vi "Day 10.vi"() -> ()   [LabVIEW 2023]
panel:
  out "Answer 2":bool[][](array[boolean])
  out "Answer 1":i32
  in  "test":bool
  in  "test input":string="addx 15\naddx -11\naddx 6\naddx -3\naddx 5\naddx -1\naddx -8\naddx 13\naddx 4\nnoop\naddx -1\naddx 5\naddx -1\naddx 5\naddx -1\naddx 5\naddx -1\naddx 5\naddx -1\naddx -35\naddx 1\naddx 24\naddx -19\naddx 1\naddx 16\naddx -11\nnoop\nnoop\naddx 21\naddx -15\nnoop\nnoop\naddx -3\naddx 9\naddx 1\naddx -3\naddx 8\naddx 1\naddx 5\nnoop\nnoop\nnoop\nnoop\nnoop\naddx -36\nnoop\naddx 1\naddx 7\nnoop\nnoop\nnoop\naddx 2\naddx 6\nnoop\nnoop\nnoop\nnoop\nnoop\naddx 1\nnoop\nnoop\naddx 7\naddx 1\nnoop\naddx -13\naddx 13\naddx 7\nnoop\naddx 1\naddx -33\nnoop\nnoop\nnoop\naddx 2\nnoop\nnoop\nnoop\naddx 8\nnoop\naddx -1\naddx 2\naddx 1\nnoop\naddx 17\naddx -9\naddx 1\naddx 1\naddx -3\naddx 11\nnoop\nnoop\naddx 1\nnoop\naddx 1\nnoop\nnoop\naddx -13\naddx -19\naddx 1\naddx 3\naddx 26\naddx -30\naddx 12\naddx -1\naddx 3\naddx 1\nnoop\nnoop\nnoop\naddx -9\naddx 18\naddx 1\naddx 2\nnoop\nnoop\naddx 9\nnoop\nnoop\nnoop\naddx -1\naddx 2\naddx -37\naddx 1\naddx 3\nnoop\naddx 15\naddx -21\naddx 22\naddx -6\naddx 1\nnoop\naddx 2\naddx 1\nnoop\naddx -10\nnoop\nnoop\naddx 20\naddx 1\naddx 2\naddx 2\naddx -6\naddx -11\nnoop\nnoop\nnoop"
  in  "input":string="noop\nnoop\nnoop\naddx 3\naddx 20\nnoop\naddx -12\nnoop\naddx 4\nnoop\nnoop\nnoop\naddx 1\naddx 2\naddx 5\naddx 16\naddx -14\naddx -25\naddx 30\naddx 1\nnoop\naddx 5\nnoop\naddx -38\nnoop\nnoop\nnoop\naddx 3\naddx 2\nnoop\nnoop\nnoop\naddx 5\naddx 5\naddx 2\naddx 13\naddx 6\naddx -16\naddx 2\naddx 5\naddx -15\naddx 16\naddx 7\nnoop\naddx -2\naddx 2\naddx 5\naddx -39\naddx 4\naddx -2\naddx 2\naddx 7\nnoop\naddx -2\naddx 17\naddx -10\nnoop\nnoop\naddx 5\naddx -1\naddx 6\nnoop\naddx -2\naddx 5\naddx -8\naddx 12\naddx 3\naddx -2\naddx -19\naddx -16\naddx 2\naddx 5\nnoop\naddx 25\naddx 7\naddx -29\naddx 3\naddx 4\naddx -4\naddx 9\nnoop\naddx 2\naddx -20\naddx 23\naddx 1\nnoop\naddx 5\naddx -10\naddx 14\naddx 2\naddx -1\naddx -38\nnoop\naddx 20\naddx -15\nnoop\naddx 7\nnoop\naddx 26\naddx -25\naddx 2\naddx 7\nnoop\nnoop\naddx 2\naddx -5\naddx 6\naddx 5\naddx 2\naddx 8\naddx -3\nnoop\naddx 3\naddx -2\naddx -38\naddx 13\naddx -6\nnoop\naddx 1\naddx 5\nnoop\nnoop\nnoop\nnoop\naddx 2\nnoop\nnoop\naddx 7\naddx 3\naddx -2\naddx 2\naddx 5\naddx 2\nnoop\naddx 1\naddx 5\nnoop\nnoop\nnoop\nnoop\nnoop\nnoop\n"
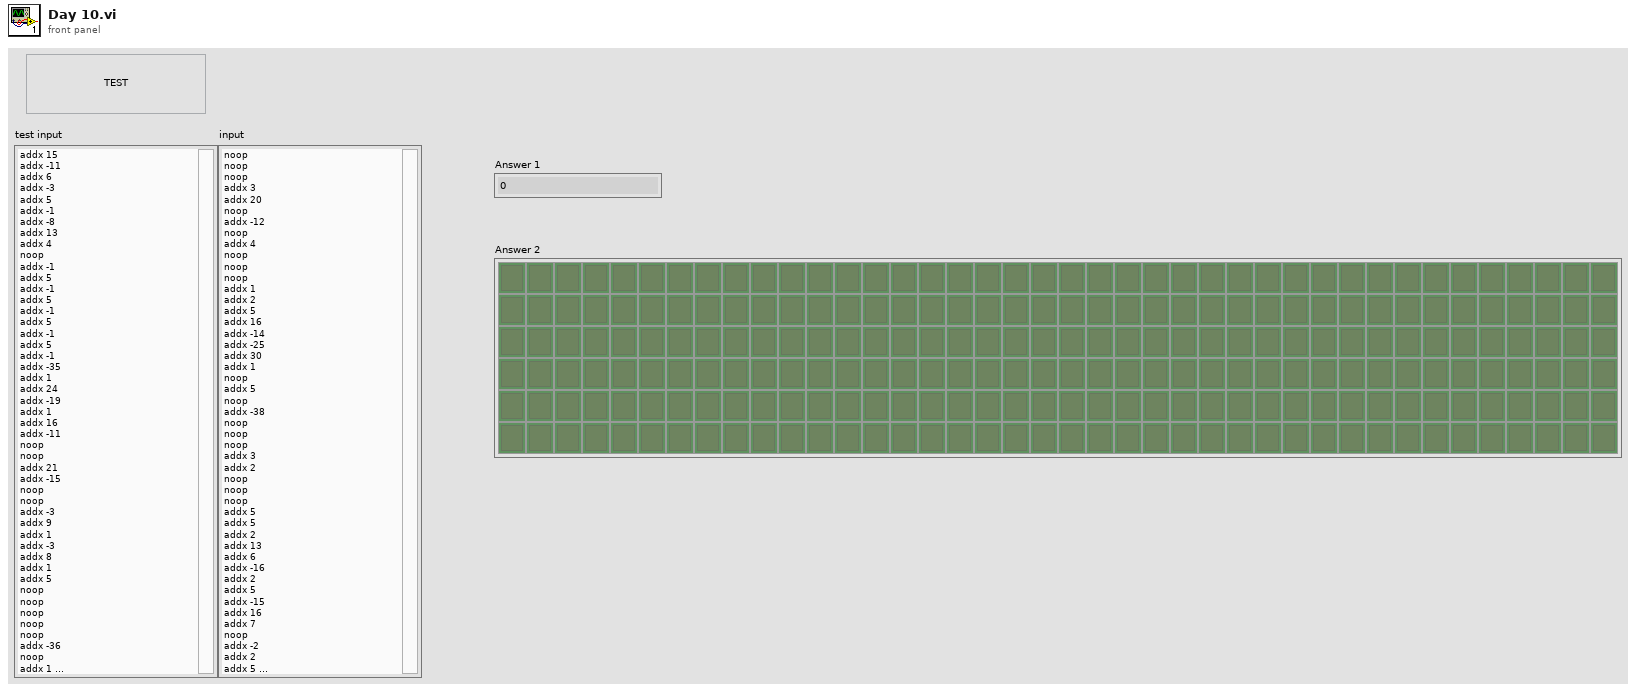
[diagram p1: front panel]
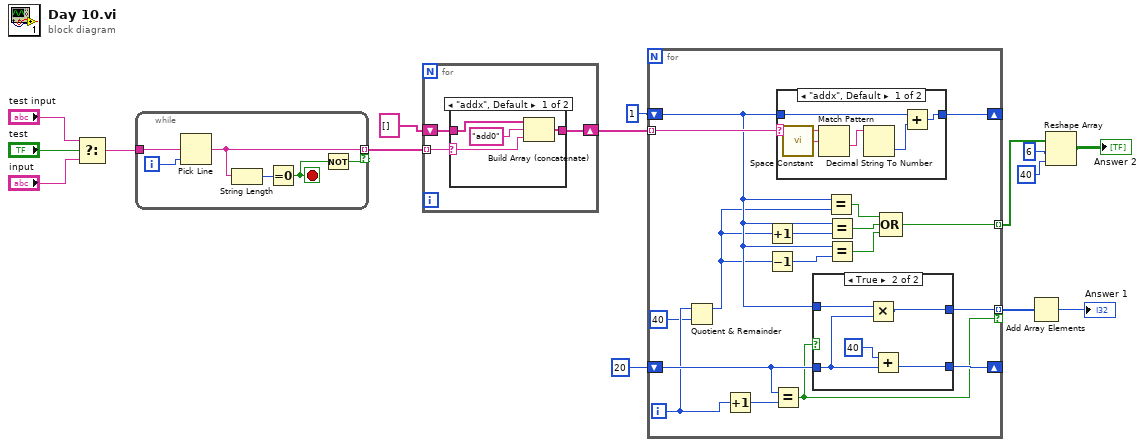
[diagram p0: block diagram]
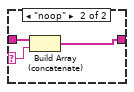
[diagram p4: hidden frame]
diagram:
  n1 = Select(t="test input", s="test", f="input") -> (s? t:f=w14:string)
  n2 = while {
    tunnel: w14 -> [w19]
    tunnel: [w18] -> w11 mode=indexing if=w16
    i -> [w20]
    stop <- w17 stop-if-true
    n3 = Pick Line(multi-line string=w19, line index=w20) -> (output string=w18:string)  [unwired: 1 in]
    n4 = String Length(string=w18) -> (length=w21:i32)
    n5 = Equal To 0?(x=w21) -> (x = 0?=w17:bool)
    n6 = Not(x=w17) -> (.not. x?=w16:bool)
  }
  n7 = for {
    tunnel: w11 -> [w24] mode=indexing
    shift-right: [w23] -> w10
    shift-left: string[] [] -> [w22]
    n8 = case shown="\"addx\", Default" w24 {
      selector: w24 -> [w28 w31]
      tunnel: [w26 w30] -> w23
      tunnel: w22 -> [w25 w29]
      frame "addx", Default {
        n9 = Build Array (concatenate)(w25, "add0" ("element"), w28) -> (w26:string[])
      }
      frame "noop" {
        n10 = Build Array (concatenate)(w29, w31) -> (w30:string[])
      }
    }
  }
  n11 = for {
    tunnel: w10 -> [w48] mode=indexing
    shift-right: [w47] -> _
    shift-left: 1 -> [w41]
    shift-right: [w46] -> _
    shift-left: 20 -> [w45]
    tunnel: [w44] -> w7 mode=indexing if=w43
    tunnel: [w36] -> w5 mode=indexing
    i -> [w34]
    n12 = Quotient & Remainder(x=w34, y=40) -> (x-y*floor(x/y)=w32:i32)  [unwired: 1 out]
    n13 = Increment(x=w34) -> (x+1=w42:i32)
    n14 = Increment(x=w32) -> (x+1=w35:i32)
    n15 = Decrement(x=w32) -> (x-1=w40:i32)
    n16 = Equal?(x=w45, y=w42) -> (x = y?=w43:bool)
    n17 = case shown="\"addx\", Default" w48 {
      selector: w48 -> [w54 _]
      tunnel: [w49 w55] -> w47
      tunnel: w41 -> [w51 w55]
      frame "addx", Default {
        n18 = call <vilib>:"Space Constant.vi"() -> ("String"=w53:string)
        n19 = Match Pattern(string=w54, regular expression=w53) -> (after substring=w52:string)  [unwired: 1 in, 3 out]
        n20 = Decimal String To Number(string=w52) -> (number=w50:i32)  [unwired: 2 in, 1 out]
        n21 = Add(x=w51, y=w50) -> (x+y=w49:i32)
      }
      frame "add0", "noop" {
      }
    }
    n22 = case shown="True" w43 {
      tunnel: [w56 w61] -> w46
      tunnel: w45 -> [w56 w58]
      tunnel: w41 -> [_ w59]
      tunnel: [_ w57] -> w44
      frame False {
      }
      frame True {
        n23 = Multiply(x=w59, y=w58) -> (x*y=w57:i32)
        n24 = Add(x=40, y=w58) -> (x+y=w61:i32)
      }
    }
    n25 = Equal?(x=w41, y=w32) -> (x = y?=w39:bool)
    n26 = Equal?(x=w41, y=w35) -> (x = y?=w38:bool)
    n27 = Equal?(x=w41, y=w40) -> (x = y?=w37:bool)
    n28 = Compound Arithmetic op=OR(w39, w38, w37) -> (w36:bool)
  }
  n29 = Add Array Elements(numeric array=w7) -> (sum=→"Answer 1":i32)
  n30 = Reshape Array(w5, 6 ("dimension size"), 40 ("dimension size")) -> (→"Answer 2":bool[][])
